vi "nanomsg_socket.vi"(4 "error in":errorcluster, 5 "linger (ms)":i32, 6 "socket type":i32(ring) items=["NN_WS"=-4, "NN_TCP"=-3, "NN_IPC"=-2, "NN_INPROC"=-1, "NN_SOL_SOCKET"=0, "NN_PAIR"=16, "NN_PUB"=32, "NN_SUB"=33, "NN_REQ"=48, "NN_REP"=49, "NN_PUSH"=80, "NN_PULL"=81, "NN_SURVEYOR"=98, "NN_RESPONDENT"=99, "NN_BUS"=112], 7 "context in":refnum<class "nanomsg_context.lvclass">) -> (0 "error out":errorcluster, 2 "socket out":refnum<class "nanomsg_socket.lvclass">, 3 "context out":refnum<class "nanomsg_context.lvclass">)   [LabVIEW 2014, in "nanomsg.lvlib" / "nanomsg_context.lvclass"]
doc: "Create a socket of flavour <b>socket type</b> in context <b>ctx in</b>.\n\nDetailed API documentation: http://nanomsg.org/documentation.html"
uses:
  nanomsg_context.lvclass
  nanomsg_socket.lvclass
  nanomsg_context.lvclass/nanomsg_context.ctl
  <vilib>/Utility/error.llb/Error Cluster From Error Code.vi
  nanomsg.lvlib
panel:
  # "NN"
  # "labview"
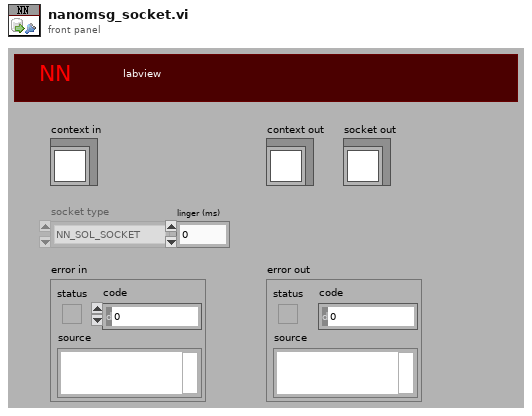
[diagram p1: front panel]
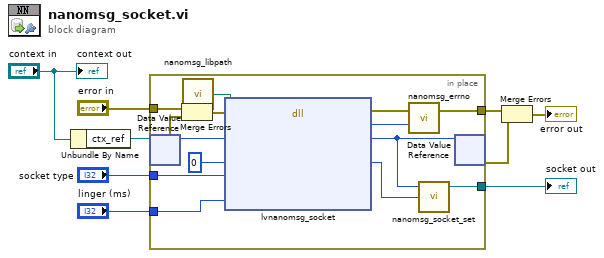
[diagram p0: block diagram]
diagram:
  n1 = Unbundle By Name("context in") -> ("ctx_ref"=w3:refnum<data-value>)
  n2 = in-place {
    in-place-border: "error in" -> [w23]
    in-place-border: "socket type" -> [w22]
    in-place-border: "linger (ms)" -> [w19]
    in-place-border: [w18] -> w5
    in-place-border: [w16] -> w4
    n3 = in-place-dvr #1(w3) -> (w15:u64, w10:errorcluster)
    n4 = Merge Errors(w23, w10) -> (w11:errorcluster)
    n5 = call "nanomsg_libpath.vi"() -> ("path"=w12:path)
    n6 = dll-call lib="?" fn="lvnanomsg_socket" ("zmq_labview.dll:lvzmq_socket")(path in=w12, error in=w11, "ctx_obj"=w15, "sock_obj"=u64 0, "type"=w22, "linger"=w19) -> (error out=w21:errorcluster, "return type"=w20:i32, "ctx_obj"=w14:u64, "sock_obj"=w17:u64)  [unwired: 3 in, 1 out]
    n7 = call "nanomsg_errno.vi"("retval"=w20, "error in"=w21) -> ("error out"=w18:errorcluster)  [unwired: 1 out]
    n8 = call "nanomsg_socket_set.vi"("socket"=w17, "context"=w14) -> ("socket out"=w16:refnum<class "nanomsg_socket.lvclass">)  [unwired: 2 in, 1 out]
    n9 = in-place-dvr #1(w14) -> (w1:errorcluster)  [unwired: 1 out]
  }
  "socket out" <- w4
  n10 = Merge Errors(w5, w1) -> (→"error out":errorcluster)
  "context out" <- "context in"
